vi "Get Measurement Details.vi"(8 "error in":errorcluster) -> (0 "error out":errorcluster, 1 "measurement annotations":T1[](array[typedef]), 2 "service class":string, 3 "measurement details":T2)   [LabVIEW 2021, in "Frequency Response_Audio ADC.lvlib"]
uses:
  Frequency Response_Audio ADC.lvlib
  <vilib>/Plug-In SDKs/Measurements/NI Measurement Plug-In SDK.lvlib
  <vilib>/gRPC/Generated APIs/ni/measurementlink/measurement/v1/RPC Messages/ni_measurementlink_measurement_v1_MeasurementDetails.ctl
  <vilib>/gRPC/Generated APIs/ni/measurementlink/measurement/v1/ni.measurementlink.measurement.v1.api.lvlib
  <vilib>/MeasurementLink/MeasurementLink Discovery Client/RPC Messages/ni_measurementlink_discovery_v1_ServiceDescriptor_AnnotationsEntry.ctl
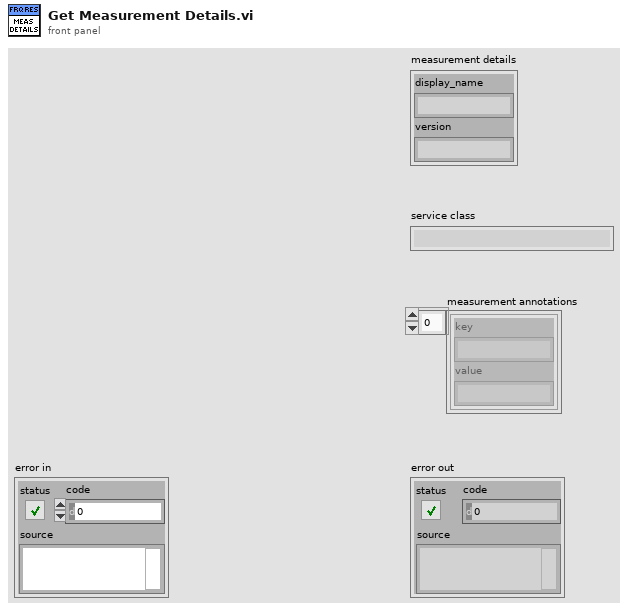
[diagram p1: front panel]
types:
  T1 = typedef "MeasurementLink Discovery Client.lvlib/ni_measurementlink_discovery_v1_ServiceDescriptor_AnnotationsEntry.ctl" = cluster{"key":string, "value":string}
  T2 = typedef "ni.measurementlink.measurement.v1.api.lvlib/ni_measurementlink_measurement_v1_MeasurementDetails.ctl" = cluster{"display_name":string, "version":string}
  T3 = typedef "NI Measurement Plug-In SDK.lvlib/Measurement Annotation.ctl" = cluster{"key":string, "value":string}
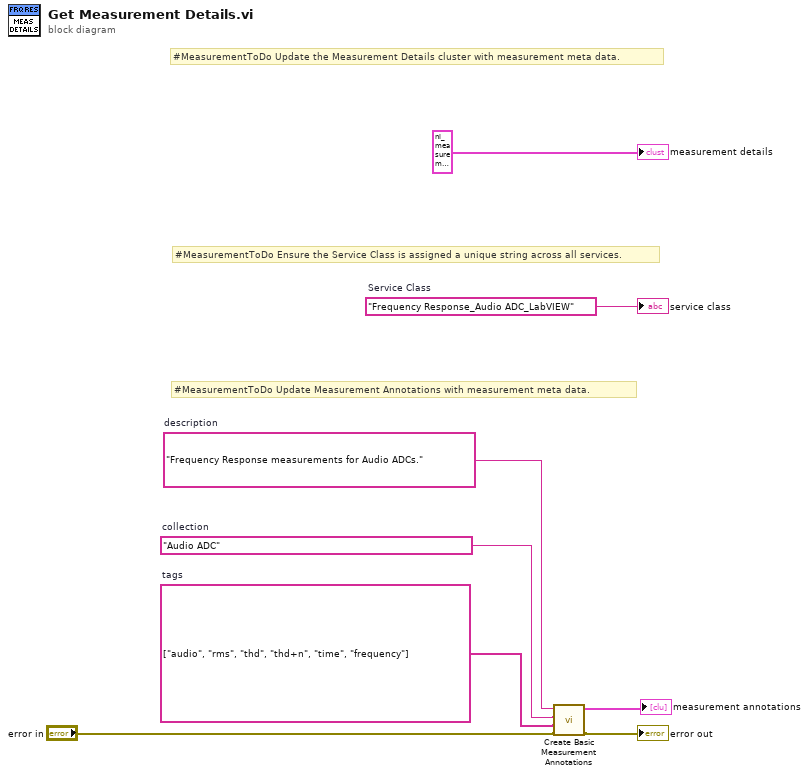
[diagram p0: block diagram]
diagram:
  w4 = string[] ["audio", "rms", "thd", "thd+n", "time", "frequency"]  # tags
  w5 = "Audio ADC"  # collection
  w6 = "Frequency Response measurements for Audio ADCs."  # description
  w8 = "Frequency Response_Audio ADC_LabVIEW"  # Service Class
  # "#MeasurementToDo Update Measurement Annotations with measurement meta data."
  # "#MeasurementToDo Ensure the Service Class is assigned a unique string across all services."
  # "#MeasurementToDo Update the Measurement Details cluster with measurement meta data."
  n1 = call <vilib>:"Create Basic Measurement Annotations.vi"("error in"="error in", "tags"=w4, "collection"=w5, "description"=w6) -> ("error out"=→"error out":errorcluster, "measurement annotations"=→"measurement annotations":T3[])  [unwired: 6 in]
  "measurement details" <- T2 {"display_name"="Frequency Response", "version"="1.0.0"} ("Measurement Details")
  "service class" <- w8
